vi "Update_Install_Path.vi"(8 "error in (no error)":errorcluster, 10 "destName":string, 11 "IB_Destination in":refnum<class "IB_Destination.lvclass">) -> (0 "error out":errorcluster, 3 "IB_Destination out":refnum<class "IB_Destination.lvclass">)   [LabVIEW 2020, in "IB_Destination.lvclass"]
uses:
  <vilib>/AppBuilder/IB_Classes/Destination/IB_Destination.lvclass
  <vilib>/AppBuilder/IB_Classes/Destination/IB_Destination.lvclass/IB_Destination.ctl
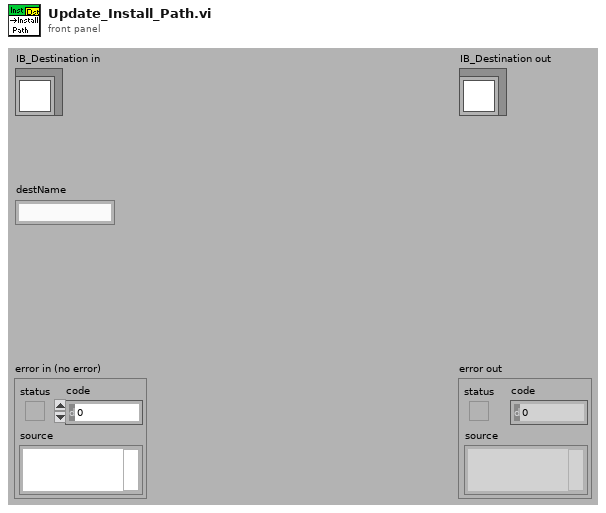
[diagram p1: front panel]
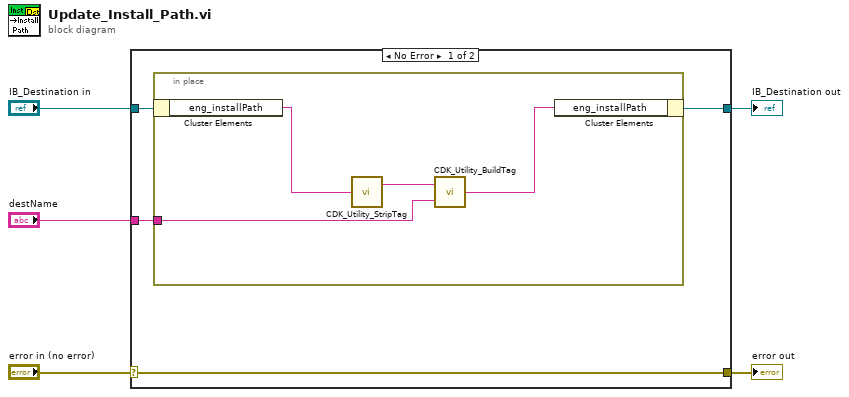
[diagram p0: block diagram]
diagram:
  n1 = case shown="No Error" "error in (no error)" {
    selector: "error in (no error)" -> [w9 w15]
    tunnel: [w9 w15] -> w4
    tunnel: [w6 w14] -> w2
    tunnel: "IB_Destination in" -> [w7 w14]
    tunnel: "destName" -> [w8 _]
    frame No Error {
      n2 = in-place {
        in-place-border: w8 -> [w12]
        n3 = in-place-cluster #1(w7) -> ("eng_installPath"=w11:string)
        n4 = call <resource>:"CDK_Utility_StripTag.vi"("Path"=w11) -> ("stripped path"=w13:string)  [unwired: 1 in, 1 out]
        n5 = call <resource>:"CDK_Utility_BuildTag.vi"("name or relative path"=w12, "BasePath"=w13) -> ("appended path"=w10:string)
        n6 = in-place-cluster #1("eng_installPath"=w10) -> (w6:refnum<class "IB_Destination.lvclass">)
      }
    }
    frame Error {
    }
  }
  "error out" <- w4
  "IB_Destination out" <- w2
